vi "英维克空调.vi"() -> ()   [LabVIEW 2016, in "环境动力监测库.lvlib" / "空调库.lvlib"]
uses:
  <vilib>/Utility/config.llb/NI_LVConfig.lvlib
panel:
  out "串口":string
  in  "查看型号":bool
  out "遥控开关机状态":bool
  in  "重开串口":bool
  in  "设定参数":bool
  in  "遥控":bool
  out "系统参数":T1
  out "告警状态":T2
  out "传感器状态":T3
  out "运行状态":T4
  out "通讯":bool
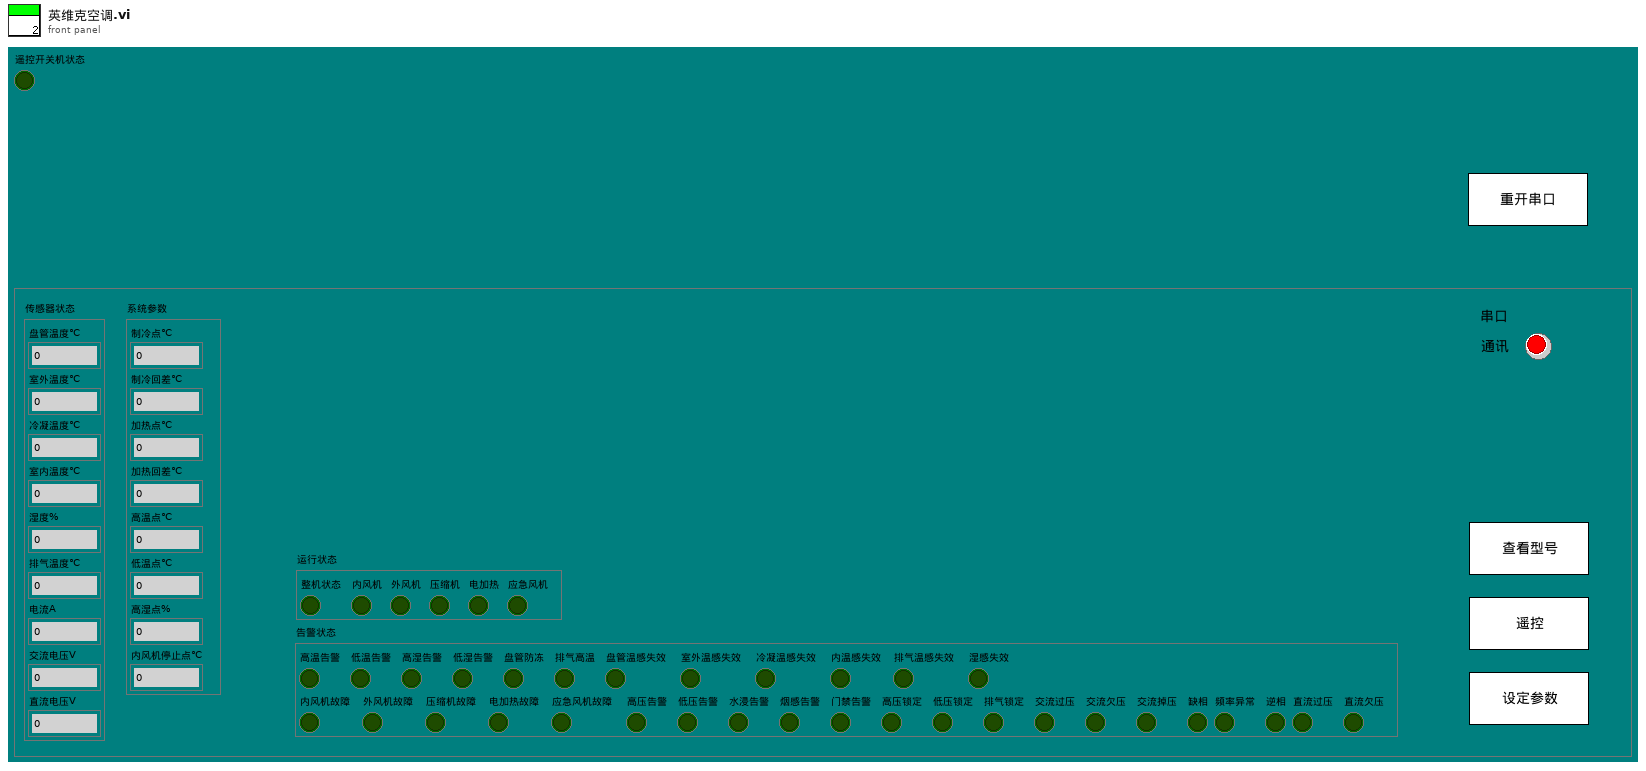
[diagram p1: front panel]
types:
  T1 = cluster{"制冷点℃":u16, "制冷回差℃":u16, "加热点℃":u16, "加热回差℃":u16, "预留":u16, "预留":u16, "高温点℃":u16, "低温点℃":u16, "高湿点%":u16, "内风机停止点℃":u16}
  T2 = cluster{"高温告警":bool, "低温告警":bool, "高湿告警":bool, "低湿告警":bool, "盘管防冻":bool, "排气高温":bool, "盘管温感失效":bool, "室外温感失效":bool, "冷凝温感失效":bool, "内温感失效":bool, "排气温感失效":bool, "湿感失效":bool, "内风机故障":bool, "外风机故障":bool, "压缩机故障":bool, "电加热故障":bool, "应急风机故障":bool, "高压告警":bool, "低压告警":bool, "水浸告警":bool, "烟感告警":bool, "门禁告警":bool, "高压锁定":bool, "低压锁定":bool, "排气锁定":bool, "交流过压":bool, "交流欠压":bool, "交流掉压":bool, "缺相":bool, "频率异常":bool, "逆相":bool, "直流过压":bool, "直流欠压":bool}
  T3 = cluster{"盘管温度℃":u16, "室外温度℃":u16, "冷凝温度℃":u16, "室内温度℃":u16, "湿度%":u16, "排气温度℃":u16, "电流A":u16, "交流电压V":u16, "直流电压V":u16}
  T4 = cluster{"整机状态":bool, "内风机":bool, "外风机":bool, "压缩机":bool, "电加热":bool, "应急风机":bool}
  T5 = typedef "NI_LVConfig.lvlib/Config Data RefNum.ctl" = refnum<k1>
  T6 = cluster{"制冷点":u16, "制冷回差":u16, "加热点":u16, "加热回差":u16, "保留":u16, "保留":u16, "高温点":u16, "低温点":u16, "高湿点":u16, "内风机停止点":u16}
  T7 = cluster{"盘管温度":u16, "室外温度":u16, "冷凝温度":u16, "室内温度":u16, "湿度":u16, "排气温度":u16, "电流":u16, "交流电压":u16, "直流电压":u16}
  T8 = cluster{"温湿度":cluster{"温度:":sgl, "状态":bool, "湿度:":sgl}, "空调":cluster{"机柜温度:":sgl, "状态":bool, "压缩机:":enum16{"停止", "运行"}, "电加热:":enum16{"停止", "运行"}}, "排气扇":cluster{"排气扇:":enum16{"关闭", "打开"}}, "冰箱":cluster{"冰箱:":enum16{"关闭", "打开"}}}
  T9 = enum16{"空调制冷点", "空调制冷回差", "加热点", "加热回差", "高温点", "低温点", "高湿点", "内风机停止点"}
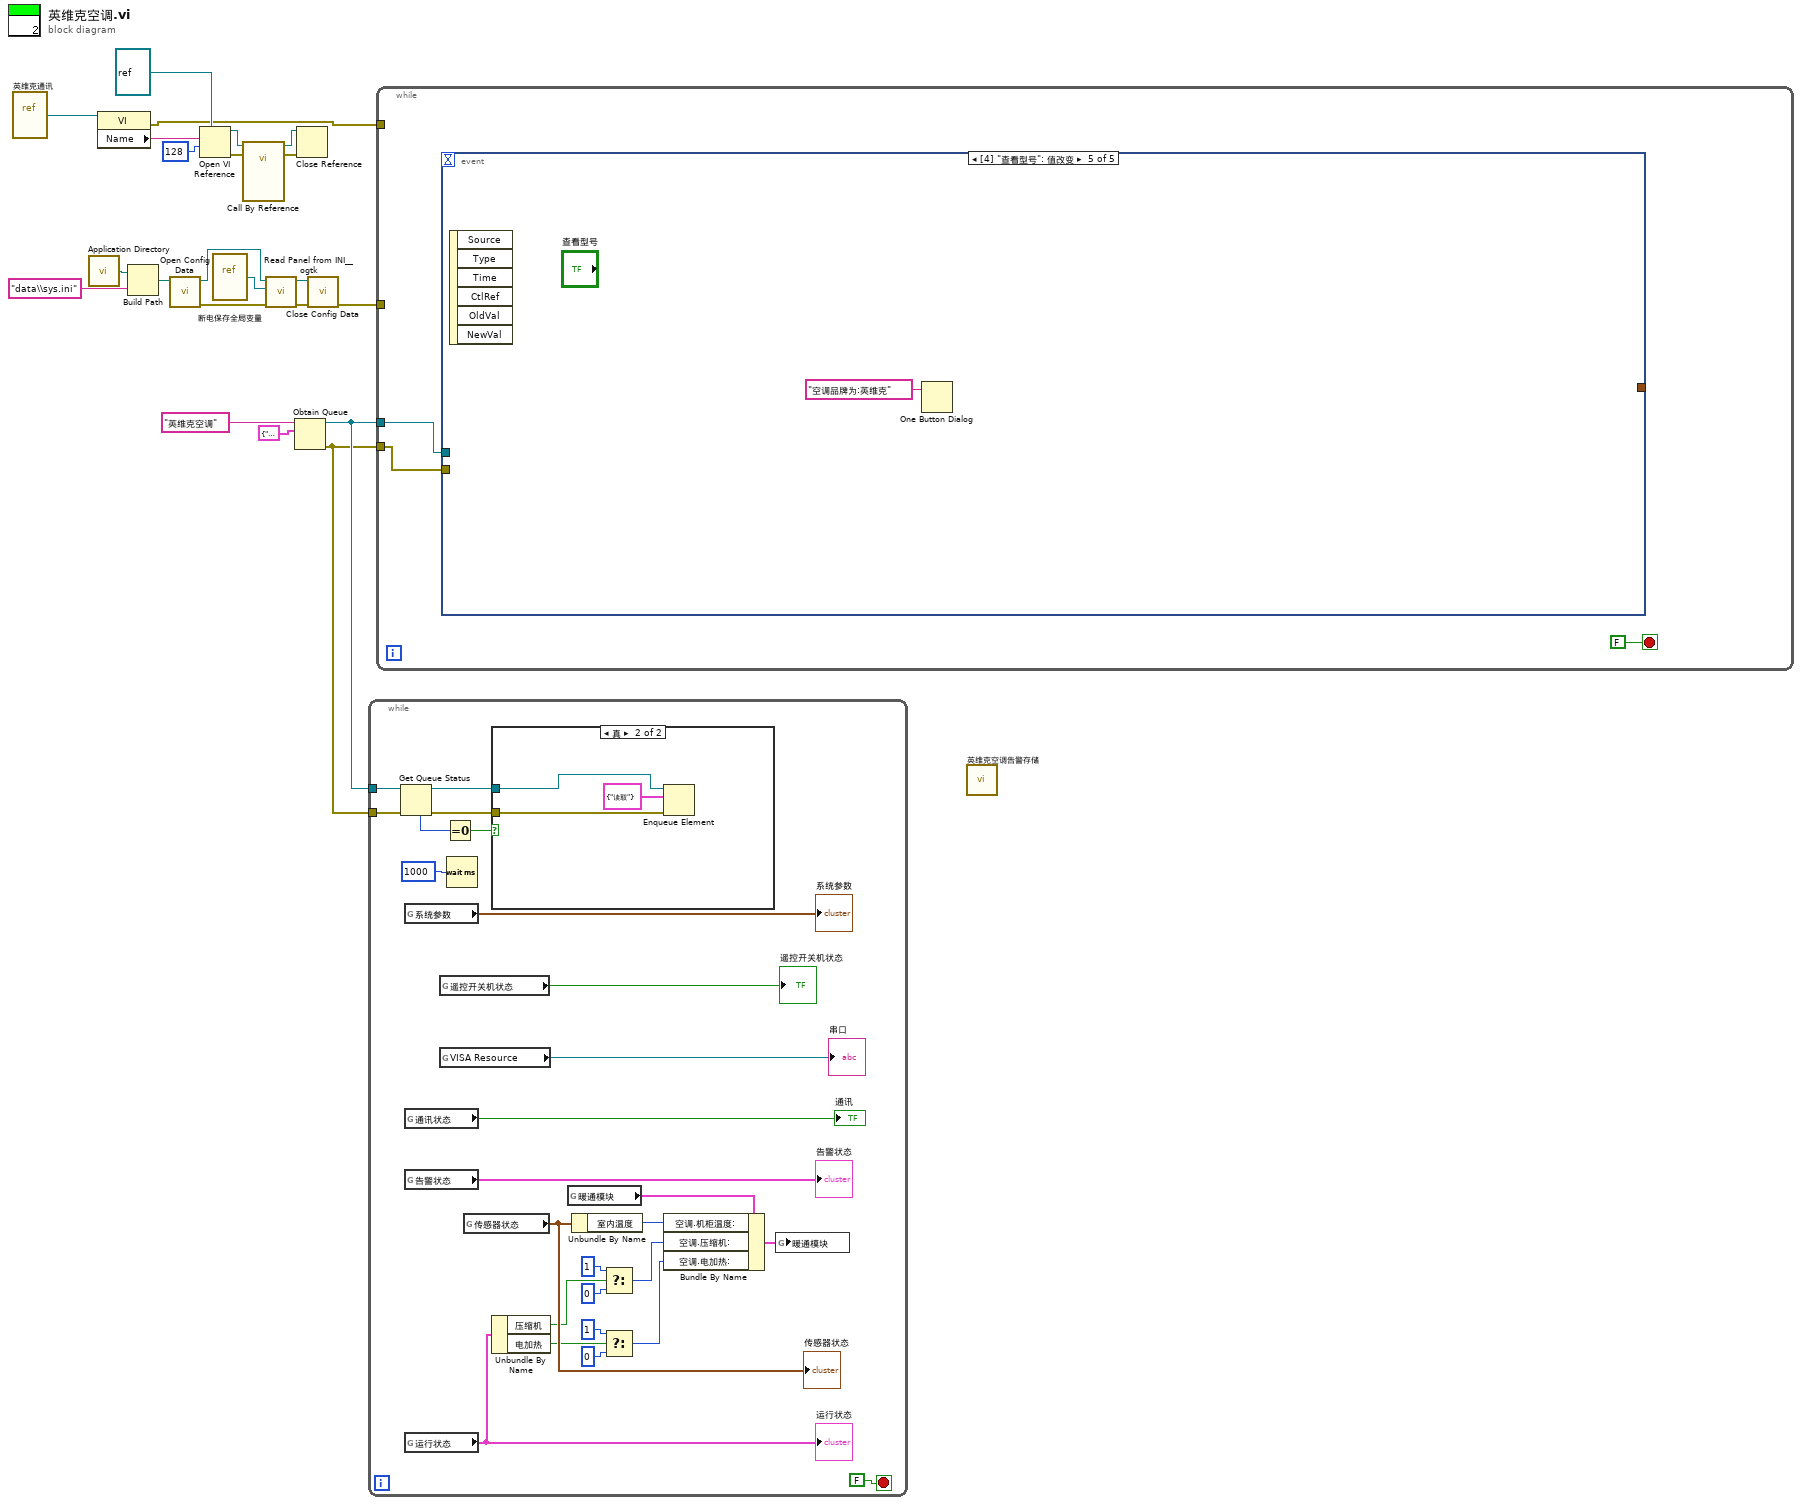
[diagram p0: block diagram]
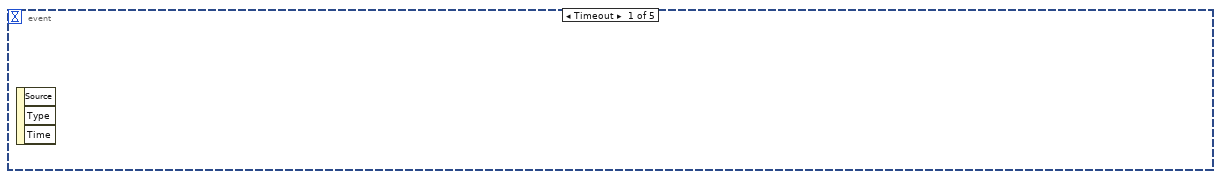
[diagram p3: hidden frame]
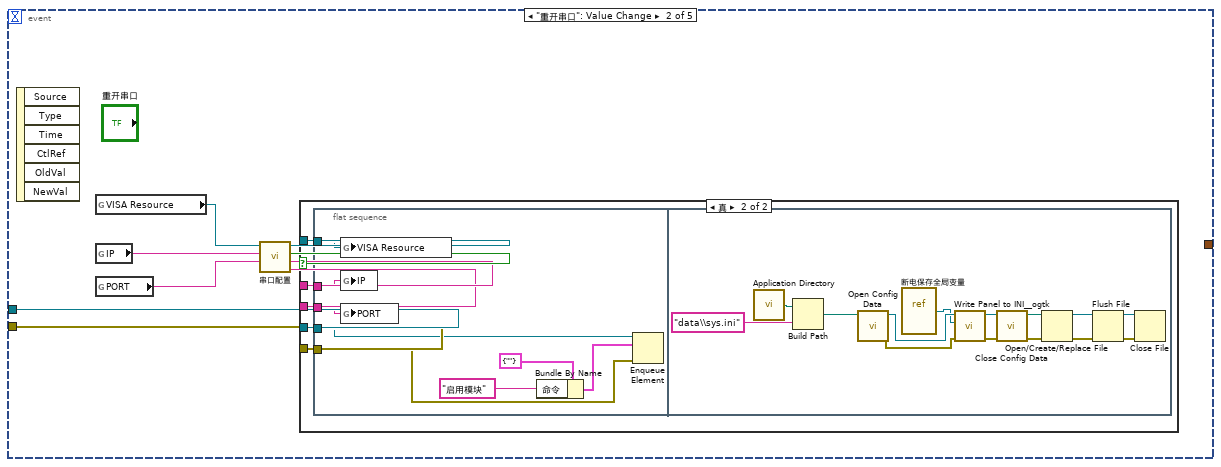
[diagram p4: hidden frame]
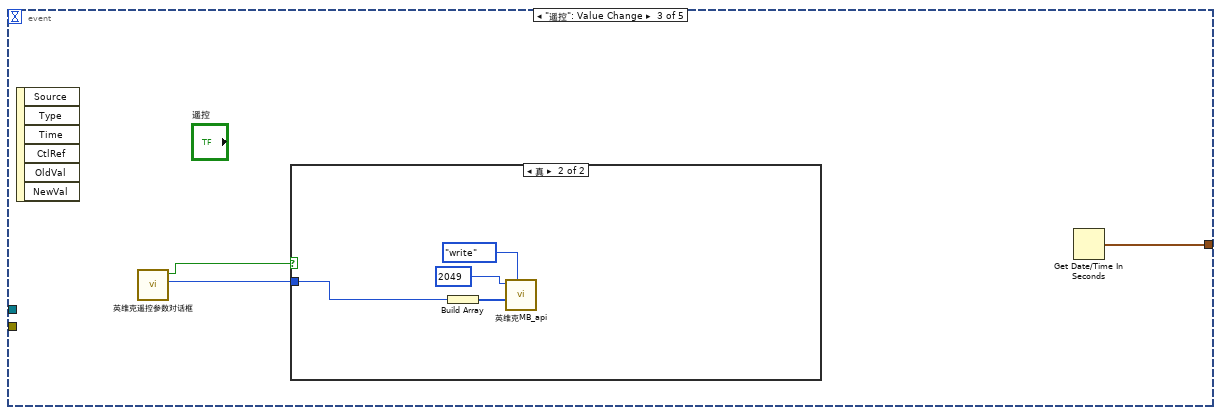
[diagram p6: hidden frame]
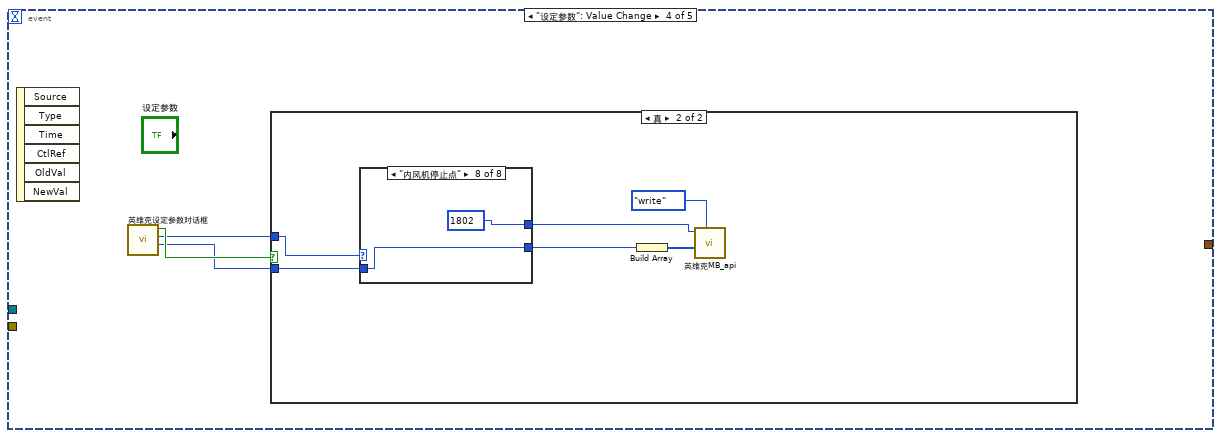
[diagram p8: hidden frame]
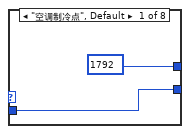
[diagram p10: hidden frame]
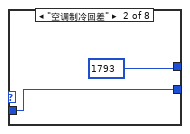
[diagram p11: hidden frame]
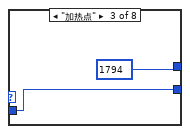
[diagram p12: hidden frame]
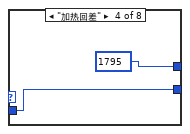
[diagram p13: hidden frame]
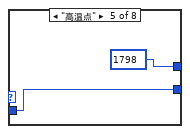
[diagram p14: hidden frame]
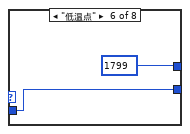
[diagram p15: hidden frame]
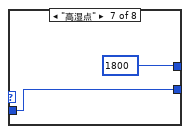
[diagram p16: hidden frame]
diagram:
  n1 = vi-ref "英维克通讯.vi"() -> (w15:refnum<vi>)
  n2 = call <vilib>:"Application Directory.vi"() -> ("Application Directory"=w14:path)
  n3 = property class="VI"(reference=w15) -> (error out=w1:errorcluster, "Name"=w16:string)  [unwired: 1 in, 1 out]
  n4 = Build Path(base path=w14, name or relative path="data\\sys.ini" ("名称或相对路径")) -> (appended path=w12:path)
  n5 = call <vilib>:"Open Config Data.vi"("configuration file path"=w12) -> ("error out"=w8:errorcluster, "refnum"=w11:T5)  [unwired: 8 in, 1 out]
  n6 = Open VI Reference(type specifier VI Refnum (for type only)=refnum<vi> refnum, vi path=w16, options=128 ("选项")) -> (vi reference=w18:refnum<vi>, error out=w20:errorcluster)  [unwired: 3 in]
  n7 = vi-ref "断电保存全局变量.vi"() -> (w10:refnum<vi>)
  n8 = call-by-ref "?"(reference=w18, error in=w20) -> (reference out=w22:refnum<vi>, error out=w21:errorcluster)  [unwired: 12 in]
  n9 = call <userlib>:"Read Panel from INI__ogtk.vi"("error in (no error)"=w8, "VI ref"=w10, "refnum"=w11) -> ("error out"=w7:errorcluster, "refnum out"=w9:T5)  [unwired: 7 in]
  n10 = Obtain Queue(name (unnamed)="英维克空调" ("名称（未命名）"), element data type=cluster{"命令":string} {"命令"="启用模块"} ("元素")) -> (queue out=w3:refnum<queue>, error out=w2:errorcluster)  [unwired: 3 in, 1 out]
  n11 = Close Reference(reference=w22, error in (no error)=w21) -> ()  [unwired: 1 out]
  n12 = call <vilib>:"Close Config Data.vi"("error in (no error)"=w7, "refnum"=w9) -> ("error out"=w6:errorcluster)  [unwired: 8 in, 1 out]
  n13 = while {
    tunnel: w3 -> [w47]
    tunnel: w2 -> [w46]
    stop <- FALSE stop-if-true
    n14 = Get Queue Status(queue=w47, error in (no error)=w46) -> (queue out=w44:refnum<queue>, error out=w43:errorcluster, # elements in queue=w48:i32)  [unwired: 1 in, 5 out]
    n15 = global read "内部交互全局变量.vi" "系统参数"() -> (→"系统参数":T6)
    n16 = global read "断电保存全局变量.vi" "通讯状态"() -> (→"通讯":bool)
    n17 = global read "内部交互全局变量.vi" "告警状态"() -> (→"告警状态":T2)
    n18 = global read "内部交互全局变量.vi" "运行状态"() -> (w31:T4)
    "运行状态" <- w31
    n19 = global read "内部交互全局变量.vi" "遥控开关机状态"() -> (→"遥控开关机状态":bool)
    n20 = global read "断电保存全局变量.vi" "VISA Resource"() -> (→"串口":refnum<visa-resource-name>)
    n21 = Equal To 0?(x=w48) -> (x = 0?=w45:bool)
    n22 = Wait (ms)(milliseconds to wait=u32 1000 ("等待时间（毫秒）")) -> ()  [unwired: 1 out]
    n23 = global read "内部交互全局变量.vi" "传感器状态"() -> (w34:T7)
    "传感器状态" <- w34
    n24 = case shown="真" w45 {
      tunnel: w44 -> [_ w51]
      tunnel: w43 -> [_ w50]
      frame False {
      }
      frame True {
        n25 = Enqueue Element(queue=w51, element=cluster{"命令":string} {"命令"="读取"} ("元素"), error in (no error)=w50) -> ()  [unwired: 1 in, 3 out]
      }
    }
    n26 = Unbundle By Name(w31) -> ("压缩机"=w30:bool, "电加热"=w25:bool)
    n27 = global read "内部交互全局变量.vi" "暖通模块"() -> (w35:T8)
    n28 = Unbundle By Name(w34) -> ("室内温度"=w33:u16)
    n29 = Select(t=1, s=w30, f=0) -> (s? t:f=w24:i32)
    n30 = Select(t=1, s=w25, f=0) -> (s? t:f=w23:i32)
    n31 = Bundle By Name(cluster=w35, "空调.机柜温度:"=w33, "空调.压缩机:"=w24, "空调.电加热:"=w23) -> (w36:T8)
    n32 = global write "内部交互全局变量.vi" "暖通模块"(w36) -> ()
  }
  n33 = while {
    tunnel: w6 -> [_]
    tunnel: w3 -> [w53]
    tunnel: w2 -> [w52]
    tunnel: w1 -> [_]
    stop <- FALSE stop-if-true
    n34 = event shown="[4] \"查看型号\": 值改变" {
      selector: _ -> [_ _ _ _ _]
      dyn-events: _ -> [_ _ _ _ _]
      timeout: _ -> [_ _ _ _ _]
      tunnel: w53 -> [_ w56 _ _ _]
      tunnel: w52 -> [_ w55 _ _ _]
      tunnel: [_ _ w91 _ _] -> _
      event Timeout {
        n35 = event-data() -> ()  [unwired: 1 in, 3 out]
      }
      event "重开串口": Value Change {
        n36 = event-data() -> ()  [unwired: 1 in, 6 out]
        n37 = global read "断电保存全局变量.vi" "VISA Resource"() -> (w63:refnum<visa-resource-name>)
        n38 = global read "断电保存全局变量.vi" "IP"() -> (w58:string)
        n39 = global read "断电保存全局变量.vi" "PORT"() -> (w57:string)
        n40 = call "串口配置.vi"("PORT"=w57, "IP"=w58, "请选择串口:"=w63) -> ("PORT 2"=w59:string, "IP 2"=w60:string, "确认 2"=w61:bool, "VISA资源名称 2"=w62:refnum<visa-resource-name>)  [unwired: 5 in]
        n41 = case shown="真" w61 {
          tunnel: w62 -> [_ w66]
          tunnel: w56 -> [_ w68]
          tunnel: w55 -> [_ w67]
          tunnel: w60 -> [_ w65]
          tunnel: w59 -> [_ w64]
          frame False {
          }
          frame True {
            n42 = flat-sequence {
              tunnel: w68 -> [w73]
              tunnel: w67 -> [w72]
              tunnel: w66 -> [w71]
              tunnel: w65 -> [w70]
              tunnel: w64 -> [w69]
              frame #0 {
                n43 = global write "断电保存全局变量.vi" "VISA Resource"(w71) -> ()
                n44 = global write "断电保存全局变量.vi" "IP"(w70) -> ()
                n45 = global write "断电保存全局变量.vi" "PORT"(w69) -> ()
                n46 = Bundle By Name(cluster=cluster{"命令":string} {"命令"=""} ("元素"), "命令"="启用模块" ("名称（未命名）")) -> (w74:cluster{"命令":string})
                n47 = Enqueue Element(queue=w73, element=w74, error in (no error)=w72) -> ()  [unwired: 1 in, 3 out]
              }
              frame #1 {
                n48 = call <vilib>:"Application Directory.vi"() -> ("Application Directory"=w89:path)
                n49 = Build Path(base path=w89, name or relative path="data\\sys.ini" ("名称或相对路径")) -> (appended path=w88:path)
                n50 = call <vilib>:"Open Config Data.vi"("configuration file path"=w88) -> ("error out"=w84:errorcluster, "refnum"=w87:T5)  [unwired: 8 in, 1 out]
                n51 = vi-ref "断电保存全局变量.vi"() -> (w86:refnum<vi>)
                n52 = call <userlib>:"Write Panel to INI__ogtk.vi"("error in (no error)"=w84, "VI ref"=w86, "refnum"=w87) -> ("error out"=w83:errorcluster, "refnum out"=w85:T5)  [unwired: 7 in]
                n53 = call <vilib>:"Close Config Data.vi"("error in (no error)"=w83, "refnum"=w85) -> ("error out"=w78:errorcluster, "file path"=w77:path)  [unwired: 8 in]
                n54 = Open/Create/Replace File(file path (use dialog)=w77, error in=w78) -> (refnum out=w81:refnum<file>, error out=w82:errorcluster)  [unwired: 4 in, 1 out]
                n55 = Flush File(refnum=w81, error in=w82) -> (refnum out=w80:refnum<file>, error out=w79:errorcluster)
                n56 = Close File(refnum=w80, error in=w79) -> ()  [unwired: 2 out]
              }
            }
          }
        }
      }
      event "遥控": Value Change {
        n57 = event-data() -> ()  [unwired: 1 in, 6 out]
        n58 = call "英维克遥控参数对话框.vi"() -> ("遥控参数选择输出"=w92:enum16{"空调关机", "空调开机"}, "确定?"=w93:bool)  [unwired: 10 in]
        n59 = case shown="真" w93 {
          tunnel: w92 -> [_ w95]
          frame False {
          }
          frame True {
            n60 = Build Array(w95) -> (w94:enum16{"空调关机", "空调开机"}[])
            n61 = call "英维克MB_api.vi"("STEP"=enum16{"open", "read", "write", "close"}."write", "values"=w94, "starting address"=u16 2049) -> ()  [unwired: 6 in, 3 out]
          }
        }
        n62 = Get Date/Time In Seconds() -> (seconds since 1Jan1904=w91:timestamp)
      }
      event "设定参数": Value Change {
        n63 = event-data() -> ()  [unwired: 1 in, 6 out]
        n64 = call "英维克设定参数对话框.vi"() -> ("参数 2"=w98:u16, "设定参数（定点数）选择 2"=w99:T9, "确定?"=w100:bool)  [unwired: 9 in]
        n65 = case shown="真" w100 {
          tunnel: w99 -> [_ w106]
          tunnel: w98 -> [_ w102]
          frame False {
          }
          frame True {
            n66 = case shown="\"内风机停止点\"" w106 {
              tunnel: [u16 1792 ("starting address") u16 1793 ("starting address") u16 1794 ("starting address") u16 1795 ("starting address") u16 1798 ("starting address") u16 1799 ("starting address") u16 1800 ("starting address") u16 1802 ("starting address")] -> w103
              tunnel: w102 -> [w107 w109 w111 w113 w115 w117 w119 w121]
              tunnel: [w107 w109 w111 w113 w115 w117 w119 w121] -> w101
              frame "空调制冷点", Default {
              }
              frame "空调制冷回差" {
              }
              frame "加热点" {
              }
              frame "加热回差" {
              }
              frame "高温点" {
              }
              frame "低温点" {
              }
              frame "高湿点" {
              }
              frame "内风机停止点" {
              }
            }
            n67 = Build Array(w101) -> (w104:u16[])
            n68 = call "英维克MB_api.vi"("STEP"=enum16{"open", "read", "write", "close"}."write", "values"=w104, "starting address"=w103) -> ()  [unwired: 6 in, 3 out]
          }
        }
      }
      event "查看型号": Value Change {
        n69 = event-data() -> ()  [unwired: 1 in, 6 out]
        n70 = One Button Dialog(message="空调品牌为:英维克" ("消息")) -> ()  [unwired: 1 in, 1 out]
      }
    }
  }
  n71 = call "英维克空调告警存储.vi"() -> ()  [unwired: 12 in]
